vi "runscenario retrieve template.vi"(6 "User Information":T2, 7 "Array":string[](array[string]), 8 "error in (no error)":errorcluster, 9 "POST (empty)":T1, 11 "Connection Refnum":T3) -> (0 "error out":errorcluster, 2 "AJAX String":string, 3 "dup Connection Refnum":T3)   [LabVIEW 2011]
uses:
  SI.LIB/ODBC/SQL Controls/Connection Refnum.ctl
  server/database/Users/User Record.ctl
  Addons/internet/utils/keyedarr.llb/Keyed Array.ctl
  OpenG.LIB/file/file.llb/Strip Path Extension - Path__ogtk.vi
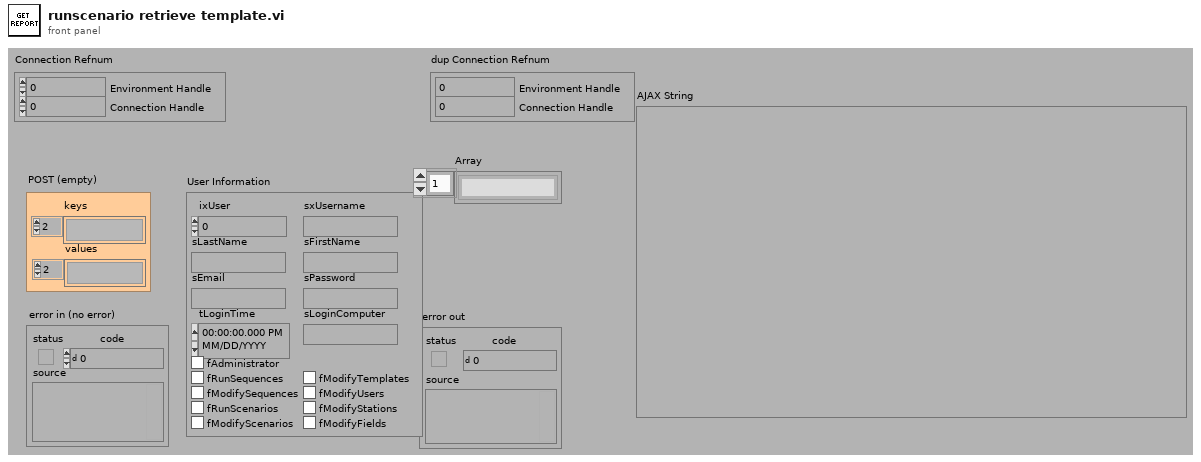
[diagram p1: front panel]
types:
  T1 = typedef "Keyed Array.ctl" = cluster{"keys":string[], "values":string[]}
  T2 = typedef "User Record.ctl" = cluster{"ixUser":i32, "sxUsername":string, "sLastName":string, "sFirstName":string, "sEmail":string, "sPassword":string, "tLoginTime":timestamp, "sLoginComputer":string, "fAdministrator":bool, "fRunSequences":bool, "fModifySequences":bool, "fRunScenarios":bool, "fModifyScenarios":bool, "fModifyTemplates":bool, "fModifyUsers":bool, "fModifyStations":bool, "fModifyFields":bool}
  T3 = typedef "Connection Refnum.ctl" = cluster{"Environment Handle":i32, "Connection Handle":i32}
  T4 = typedef "Datasheet Report Info.ctl" = cluster{"sxTemplateId":string[], "reportPath":path}
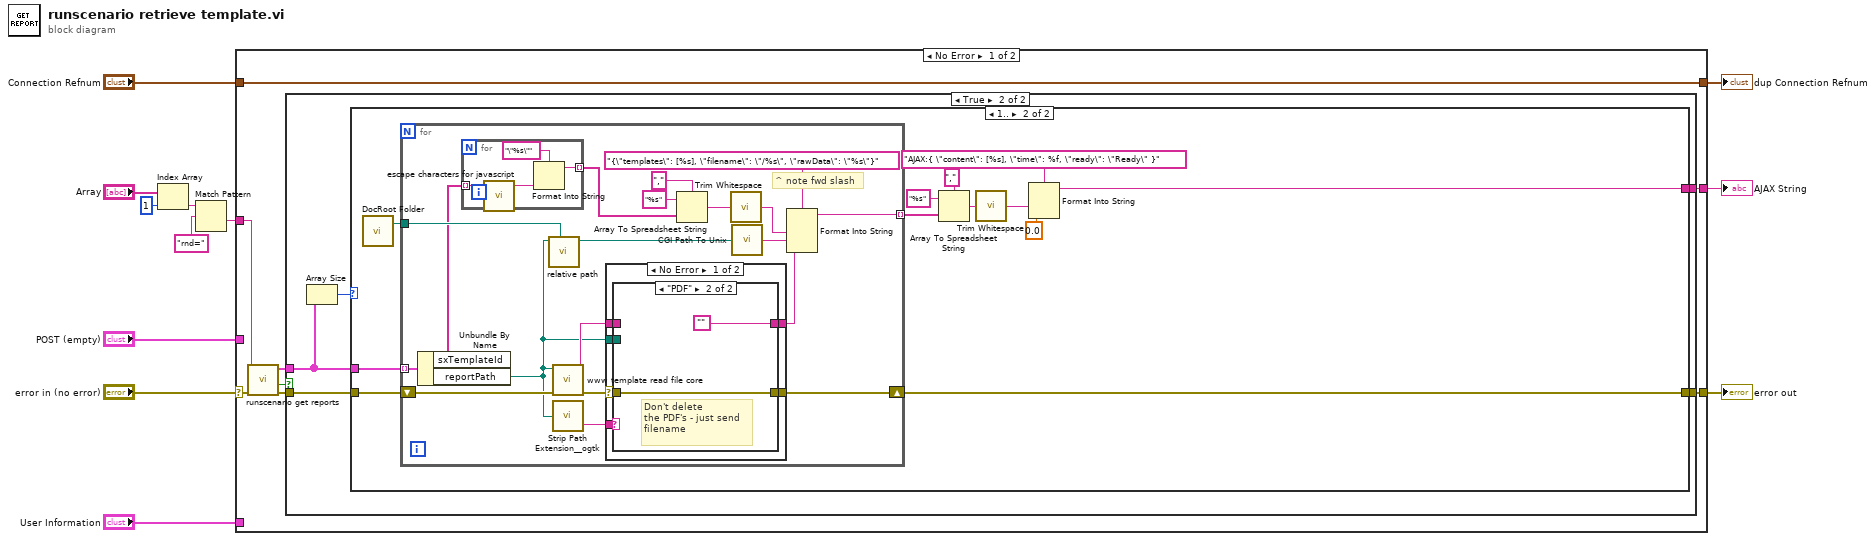
[diagram p0: block diagram]
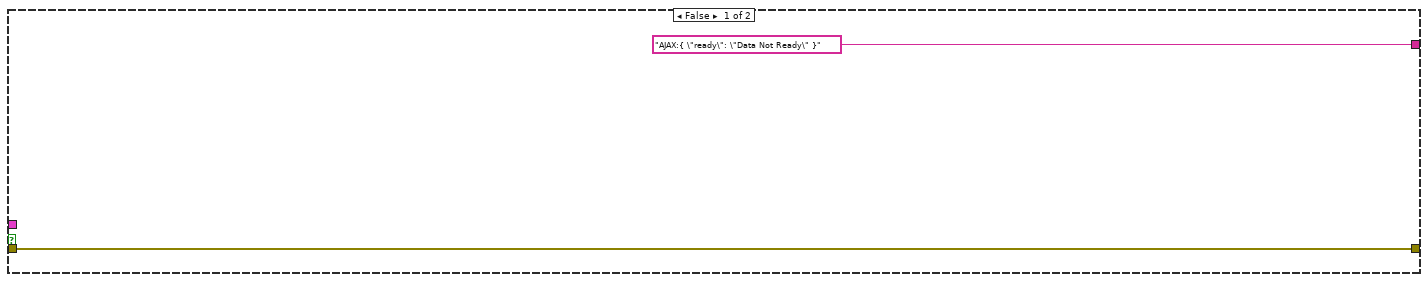
[diagram p2: hidden frame]
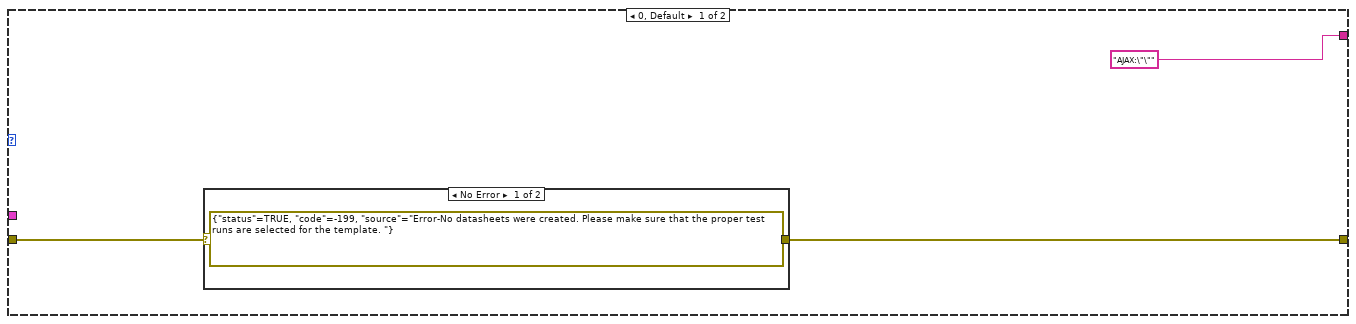
[diagram p3: hidden frame]
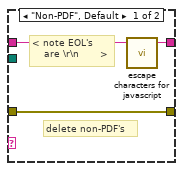
[diagram p5: hidden frame]
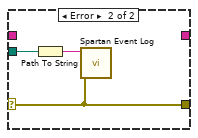
[diagram p6: hidden frame]
diagram:
  n1 = Index Array(array="Array", index=1) -> (element=w5:string)
  n2 = Match Pattern(string=w5, regular expression="rnd=" ("format string")) -> (after substring=w2:string)  [unwired: 1 in, 3 out]
  n3 = case shown="No Error" "error in (no error)" {
    selector: "error in (no error)" -> [w18 w82]
    tunnel: "Connection Refnum" -> [w20 w83]
    tunnel: [w19 w82] -> w11
    tunnel: "User Information" -> [_ _]
    tunnel: "POST (empty)" -> [_ _]
    tunnel: [w20 w83] -> w8
    tunnel: w2 -> [w14 _]
    tunnel: [w13 _] -> w1
    frame No Error {
      n4 = call "runscenario get reports.vi"("error in (no error)"=w18, "jobid"=w14) -> ("error out"=w17:errorcluster, "READY?"=w15:bool, "Datasheet Paths"=w16:T4[])  [unwired: 7 in]
      n5 = case shown="True" w15 {
        tunnel: ["AJAX:{ \"ready\": \"Data Not Ready\" }" w25] -> w13
        tunnel: [w22 w27] -> w19
        tunnel: w17 -> [w22 w26]
        tunnel: w16 -> [_ w23]
        frame False {
        }
        frame True {
          n6 = Array Size(array=w23) -> (size(s)=w24:i32)
          n7 = case shown="1.." w24 {
            tunnel: [w30 w40] -> w27
            tunnel: w26 -> [w28 w39]
            tunnel: w23 -> [_ w38]
            tunnel: ["AJAX:\"\"" w34] -> w25
            frame 0, Default {
              n8 = case shown="No Error" w28 {
                selector: w28 -> [_ w32]
                tunnel: [errorcluster {"status"=TRUE, "code"=-199, "source"="Error-No datasheets were created. Please make sure that the proper test runs are selected for the template. "} ("error out") w32] -> w30
                frame No Error {
                }
                frame Error {
                }
              }
            }
            frame 1.. {
              n9 = call "DocRoot Folder.vi"() -> ("DocumentRoot Folder"=w33:path)  [unwired: 3 in]
              n10 = for {
                shift-right: [w47] -> w40
                shift-left: w39 -> [w63]
                tunnel: [w61] -> w44 mode=indexing
                tunnel: w33 -> [w57]
                tunnel: w38 -> [w56] mode=indexing
                # "^ note fwd slash"
                n11 = Unbundle By Name(w56) -> ("sxTemplateId"=w54:string[], "reportPath"=w55:path)
                n12 = for {
                  tunnel: w54 -> [w81] mode=indexing
                  tunnel: [w78] -> w53 mode=indexing
                  n13 = call "escape characters for javascript.vi"("String (\"\")"=w81) -> ("escaped String"=w80:string)  [unwired: 4 out]
                  n14 = Format Into String(format string="\"%s\"", w80) -> (resulting string=w78:string)  [unwired: 2 in, 1 out]
                }
                n15 = call "relative path.vi"("Base Path (empty)"=w57, "Absolute Path (empty)"=w55) -> ("Path Relative to Base"=w46:path)  [unwired: 3 out]
                n16 = call "www template read file core.vi"("error in (no error)"=w63, "Path"=w55) -> ("error out"=w45:errorcluster, "File Content"=w60:string)  [unwired: 8 out]
                n17 = call-poly "Strip Path Extension__ogtk.vi"("path"=w55) -> ("extension"=w58:string)  [unwired: 1 out]
                n18 = case shown="No Error" w45 {
                  selector: w45 -> [w64 w77]
                  tunnel: w60 -> [w69 _]
                  tunnel: [w68 _] -> w59
                  tunnel: w58 -> [w67 _]
                  tunnel: w55 -> [w66 w76]
                  tunnel: [w65 w77] -> w47
                  frame No Error {
                    n19 = case shown="\"PDF\"" w67 {
                      tunnel: [w70 w73] -> w65
                      tunnel: w64 -> [w70 w73]
                      tunnel: w66 -> [_ _]
                      tunnel: w69 -> [w72 _]
                      tunnel: [w71 ""] -> w68
                      frame "Non-PDF", Default {
                        # "< note EOL's\n    are \\r\\n       >"
                        # "delete non-PDF's"
                        n20 = call "escape characters for javascript.vi"("String (\"\")"=w72) -> ("escaped String"=w71:string)  [unwired: 4 out]
                      }
                      frame "PDF" {
                        # "Don't delete\nthe PDF's - just send\nfilename"
                      }
                    }
                  }
                  frame Error {
                    n21 = Path To String(path=w76) -> (string=w75:string)
                    n22 = call "Spartan Event Log.vi"("error in (no error)"=w77, "message (\"\")"=w75) -> ()  [unwired: 6 in, 1 out]
                  }
                }
                n23 = Array To Spreadsheet String(delimiter (Tab)="," ("format string"), array=w53, 3:"%s" ("format string")) -> (spreadsheet string=w50:string)
                n24 = call <vilib>:"Trim Whitespace.vi"("string"=w50) -> ("trimmed string"=w49:string)  [unwired: 1 in]
                n25 = call "CGI Path To Unix.vi"("platform path"=w46) -> ("unix path"=w48:string)  [unwired: 1 in]
                n26 = Format Into String(format string="{\"templates\": [%s], \"filename\": \"/%s\", \"rawData\": \"%s\"}", w49, w48, w59) -> (resulting string=w61:string)  [unwired: 2 in, 1 out]
              }
              n27 = Array To Spreadsheet String(delimiter (Tab)=",", array=w44, 3:"%s") -> (spreadsheet string=w41:string)
              n28 = call <vilib>:"Trim Whitespace.vi"("string"=w41) -> ("trimmed string"=w35:string)  [unwired: 1 in]
              n29 = Format Into String(format string="AJAX:{ \"content\": [%s], \"time\": %f, \"ready\": \"Ready\" }" ("Template (\"\")"), w35, 0.0 ("input 2")) -> (resulting string=w34:string)  [unwired: 2 in, 1 out]
            }
          }
        }
      }
    }
    frame Error {
    }
  }
  "dup Connection Refnum" <- w8
  "error out" <- w11
  "AJAX String" <- w1
